vi "FLSBP1006_加时序.vi"() -> ()   [LabVIEW 2016]
uses:
  <vilib>/Instr/_visa.llb/VISA Configure Serial Port (Instr).vi
panel:
  out "命令显示":string
  in  "复位":bool
  in  "暂停":bool
  in  "小数":string
  in  "卡滞发生时间":string
  in  "角度（小数）":string
  in  "卡滞角度":string
  in  "退化故障":string(combo)
  in  "控制方法":string(combo)
  out "Pitch":dbl(graph)
  out "Roll":dbl(graph)
  in  "波特率":dbl=115200.0
  in  "故障腿":string(combo)
  in  "data bits (8)":u16=8 caption="数据比特(8)" min=5 max=8 step=1
  in  "arduino端口":refnum<visa-resource-name>
  in  "控制程序启动":bool
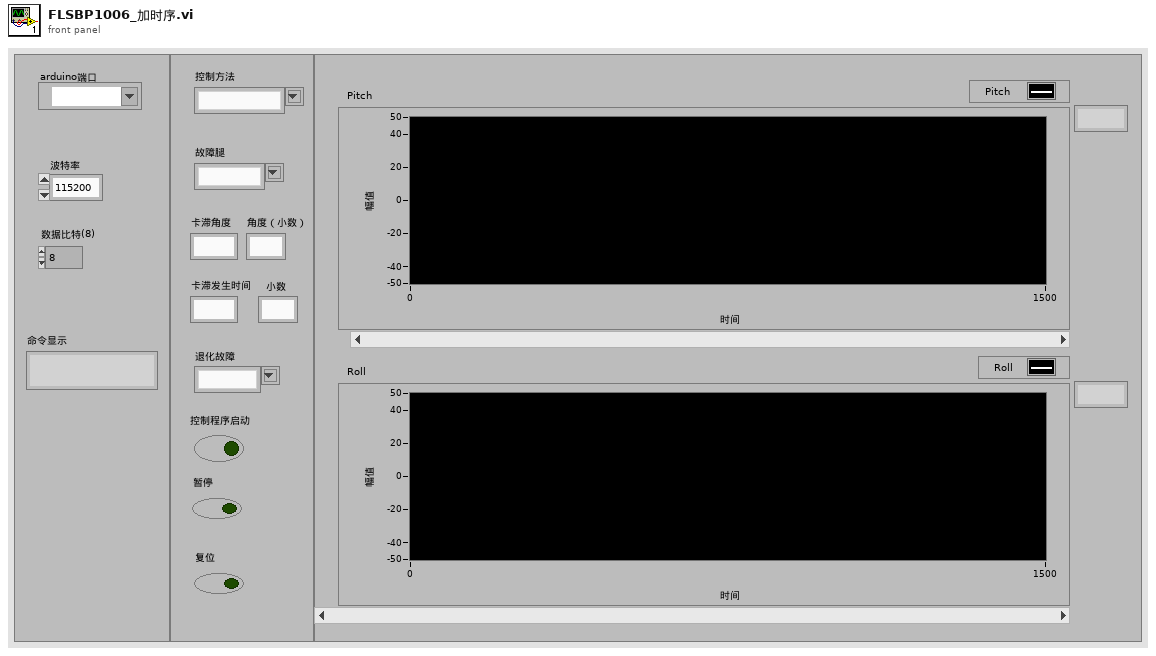
[diagram p1: front panel]
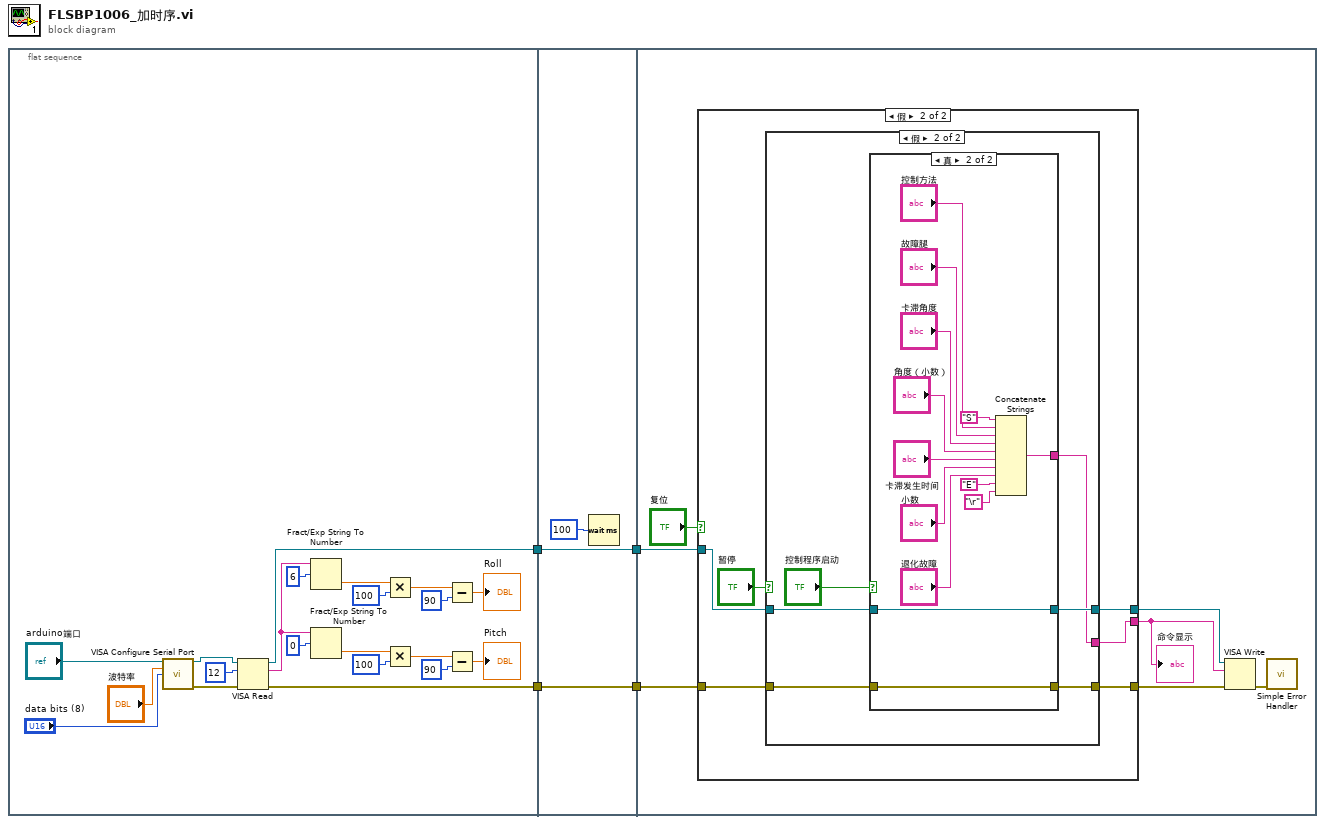
[diagram p0: block diagram]
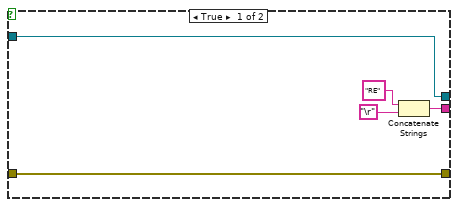
[diagram p2: hidden frame]
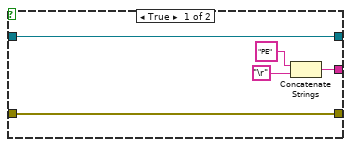
[diagram p3: hidden frame]
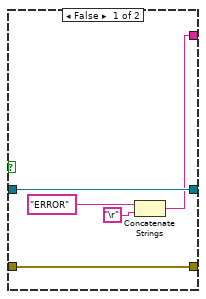
[diagram p4: hidden frame]
diagram:
  n1 = flat-sequence {
    tunnel: [w7] -> w4
    tunnel: [w5] -> w3
    tunnel: w4 -> [w28]
    tunnel: w3 -> [w27]
    tunnel: [w28] -> w2
    tunnel: [w27] -> w1
    tunnel: w2 -> [w30]
    tunnel: w1 -> [w29]
    frame #0 {
      n2 = call-poly "VISA Configure Serial Port"("VISA resource name"="arduino端口", "baud rate (9600)"="波特率", "data bits (8)"="data bits (8)") -> ("VISA resource name out"=w22:refnum<visa-resource-name>, "error out"=w6:errorcluster)  [unwired: 11 in]
      n3 = VISA Read(VISA resource name=w22, byte count=12, error in (no error)=w6) -> (VISA resource name out=w7:refnum<visa-resource-name>, read buffer=w10:string, error out=w5:errorcluster)  [unwired: 1 out]
      n4 = Fract/Exp String To Number(string=w10, offset=6) -> (number=w14:dbl)  [unwired: 3 out]
      n5 = Fract/Exp String To Number(string=w10, offset=0) -> (number=w19:dbl)  [unwired: 3 out]
      n6 = Multiply(x=w14, y=100) -> (x*y=w12:dbl)
      n7 = Multiply(x=w19, y=100) -> (x*y=w17:dbl)
      n8 = Subtract(x=w12, y=90) -> (x-y=→"Roll":dbl)
      n9 = Subtract(x=w17, y=90) -> (x-y=→"Pitch":dbl)
    }
    frame #1 {
      n10 = Wait (ms)(milliseconds to wait=u32 100 ("等待时间（毫秒）")) -> ()  [unwired: 1 out]
    }
    frame #2 {
      n11 = case shown="假" "复位" {
        tunnel: w30 -> [w36 w46]
        tunnel: w29 -> [w37 w45]
        tunnel: [w36 w43] -> w33
        tunnel: [w38 w42] -> w35
        tunnel: [w37 w41] -> w34
        frame True {
          n12 = Concatenate Strings("RE", "\r") -> (w38:string)
        }
        frame False {
          n13 = case shown="假" "暂停" {
            tunnel: w46 -> [w49 w57]
            tunnel: w45 -> [w47 w55]
            tunnel: [w49 w54] -> w43
            tunnel: [w48 w53] -> w42
            tunnel: [w47 w52] -> w41
            frame True {
              n14 = Concatenate Strings("PE", "\r") -> (w48:string)
            }
            frame False {
              n15 = case shown="真" "控制程序启动" {
                tunnel: w57 -> [w61 w65]
                tunnel: w55 -> [w62 w63]
                tunnel: [w61 w65] -> w54
                tunnel: [w58 w64] -> w53
                tunnel: [w62 w63] -> w52
                frame False {
                  n16 = Concatenate Strings("ERROR", "\r") -> (w58:string)
                }
                frame True {
                  n17 = Concatenate Strings("S", "控制方法", "故障腿", "卡滞角度", "角度（小数）", "卡滞发生时间", "小数", "退化故障", "E", "\r") -> (w64:string)
                }
              }
            }
          }
        }
      }
      "命令显示" <- w35
      n18 = VISA Write(VISA resource name=w33, write buffer=w35, error in (no error)=w34) -> (error out=w32:errorcluster)  [unwired: 2 out]
      n19 = call <vilib>:"Simple Error Handler.vi"("error in (no error)"=w32) -> ()  [unwired: 1 in, 8 out]
    }
  }
